vi "Write_tcpClientQueueFromDds.vi"(8 "error in (no error)":errorcluster, 10 "tcpClientQueueFromDds":refnum<queue>, 11 "TcpServerTel in":refnum<class "TcpServerTel.lvclass">) -> (0 "error out":errorcluster, 3 "TcpServerTel out":refnum<class "TcpServerTel.lvclass">)   [LabVIEW 2018, in "TcpServerTel.lvclass"]
doc: "Write the ttcpClientQueueFromDds."
uses:
  TcpServerTel.lvclass
  TcpServerTel.lvclass/TcpServerTel.ctl
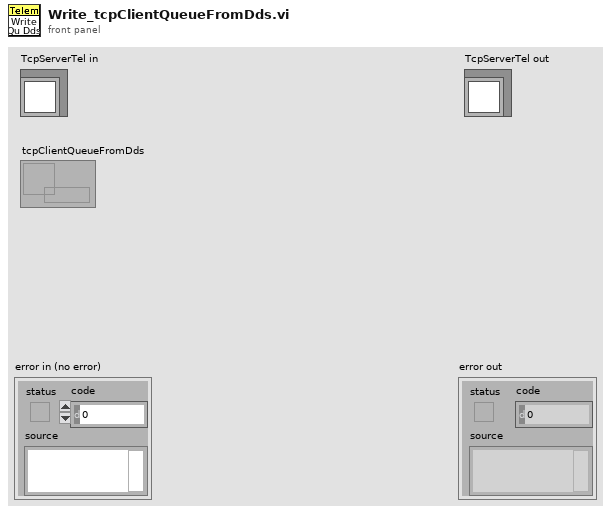
[diagram p1: front panel]
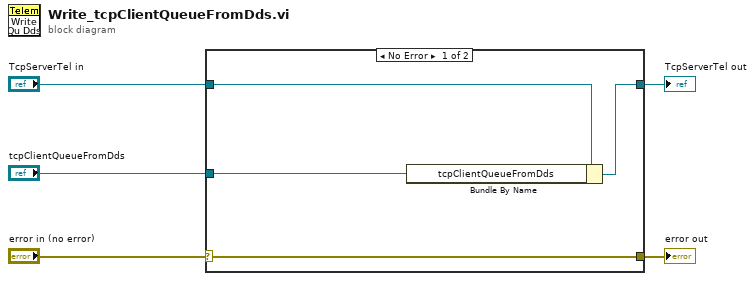
[diagram p0: block diagram]
diagram:
  n1 = case shown="No Error" "error in (no error)" {
    selector: "error in (no error)" -> [w9 w10]
    tunnel: [w9 w10] -> w4
    tunnel: [w7 w11] -> w2
    tunnel: "TcpServerTel in" -> [w8 w11]
    tunnel: "tcpClientQueueFromDds" -> [w6 _]
    frame No Error {
      n2 = Bundle By Name(cluster=w8, "tcpClientQueueFromDds"=w6) -> (w7:refnum<class "TcpServerTel.lvclass">)
    }
    frame Error {
    }
  }
  "error out" <- w4
  "TcpServerTel out" <- w2
